vi "GetDefaultConfigFilePath.vi"(8 "error in (no error)":errorcluster, 11 "Device in":refnum<class "Device.lvclass">) -> (0 "error out":errorcluster, 2 "Path":path, 3 "Device out":refnum<class "Device.lvclass">)   [LabVIEW 2020, in "Device.lvlib" / "Device.lvclass"]
uses:
  Device.lvclass
  Device.lvclass/Device.ctl
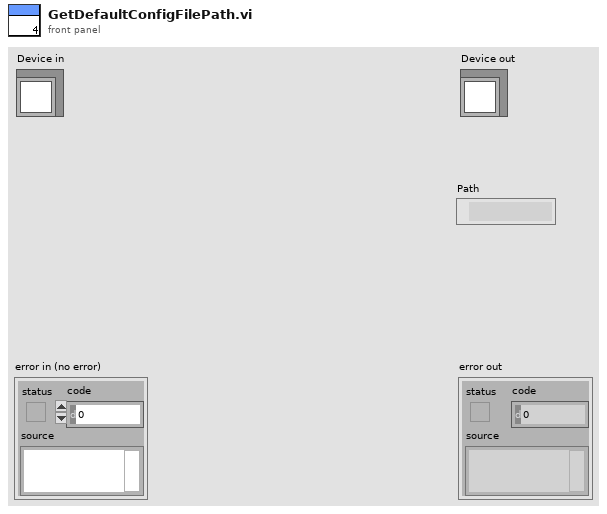
[diagram p1: front panel]
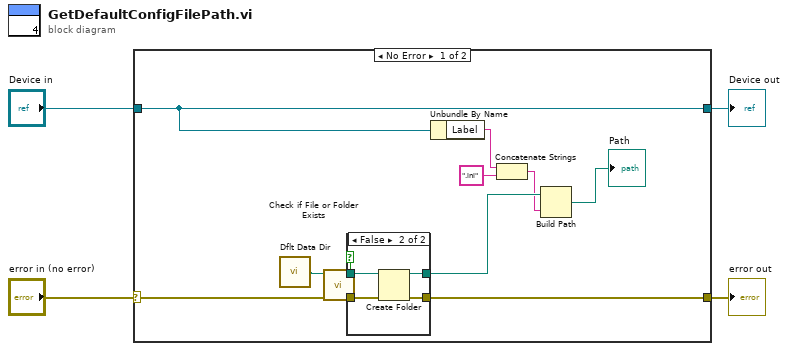
[diagram p0: block diagram]
diagram:
  n1 = case shown="No Error" "error in (no error)" {
    selector: "error in (no error)" -> [w11 w24]
    tunnel: [w10 w24] -> w3
    tunnel: [w8 w23] -> w1
    tunnel: "Device in" -> [w8 w23]
    frame No Error {
      n2 = call <vilib>:"Dflt Data Dir.vi"() -> ("App:Default Data Directory"=w13:path)
      n3 = call <vilib>:"Check if File or Folder Exists.vi"("error in (no error)"=w11, "path"=w13) -> ("error out"=w15:errorcluster, "file or folder exists?"=w14:bool, "dup path"=w16:path)  [unwired: 7 in]
      n4 = case shown="False" w14 {
        tunnel: w15 -> [w17 w22]
        tunnel: w16 -> [w18 w21]
        tunnel: [w17 w20] -> w10
        tunnel: [w18 w19] -> w12
        frame True {
        }
        frame False {
          n5 = Create Folder(path (use dialog)=w21, error in=w22) -> (created path=w19:path, error out=w20:errorcluster)  [unwired: 1 in, 1 out]
        }
      }
      n6 = Unbundle By Name(w8) -> ("Label"=w7:string)
      n7 = Concatenate Strings(w7, ".ini" ("string")) -> (w5:string)
      n8 = Build Path(base path=w12, name or relative path=w5) -> (appended path=→"Path":path)
    }
    frame Error {
    }
  }
  "error out" <- w3
  "Device out" <- w1
